vi "RemotePanel.vi"(0 "Refresh":i32=250, 1 "Remote Path":path, 2 "Remote App":refnum<vi>, 3 "Local  VI":refnum<vi>) -> ()   [LabVIEW 2014]
panel:
  out "Label.Text":string
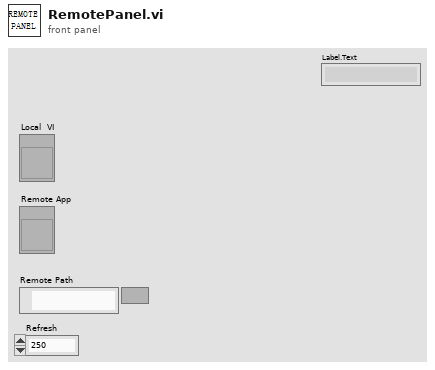
[diagram p1: front panel]
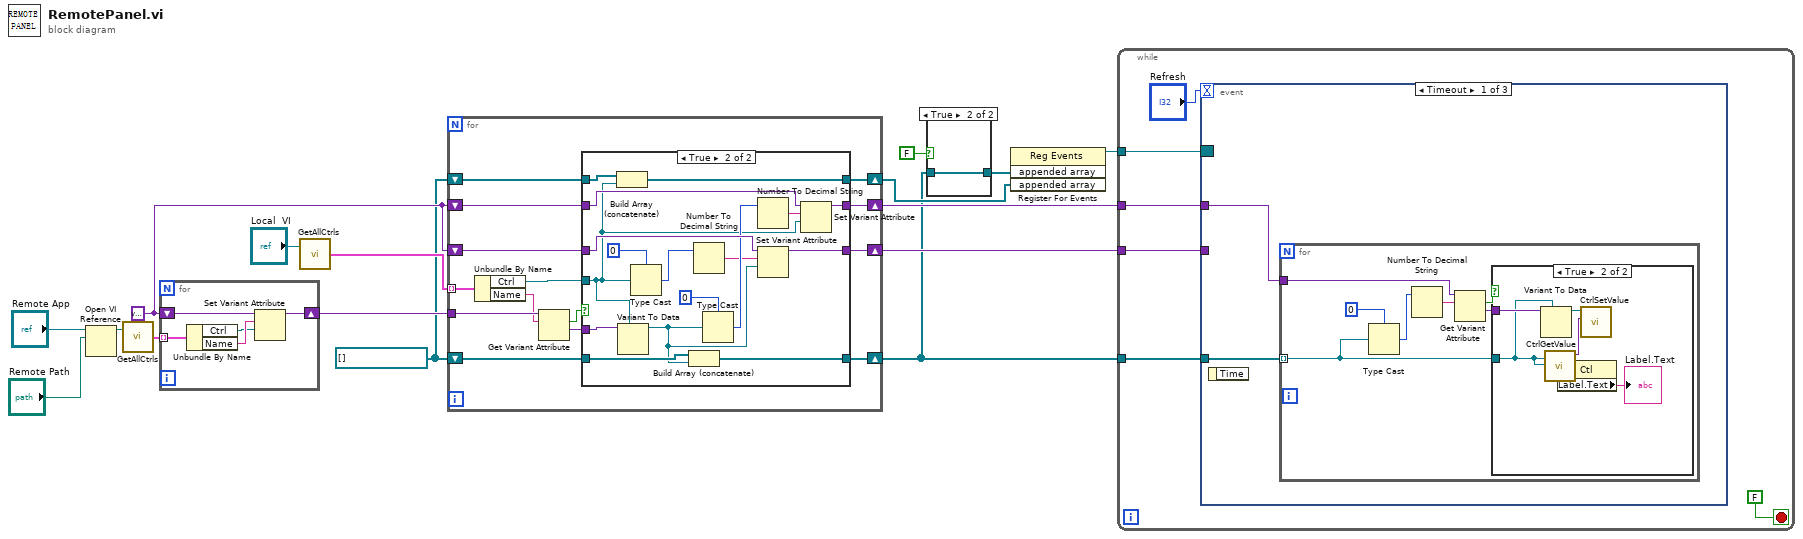
[diagram p0: block diagram]
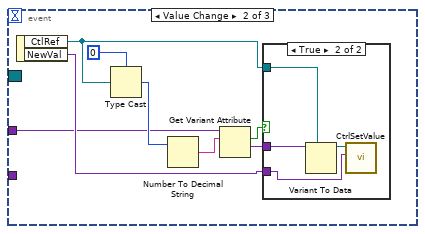
[diagram p5: hidden frame]
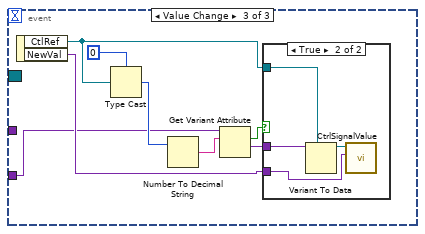
[diagram p7: hidden frame]
diagram:
  w9 = refnum<vi>[] [] ("appended array")
  w10 = variant ("variant")
  n1 = Open VI Reference(application reference (local)="Remote App", vi path="Remote Path") -> (vi reference=w13:refnum<vi>)  [unwired: 4 in, 1 out]
  n2 = call "GetAllCtrls.vi"("VI"=w13) -> ("Ctrls"=w14:cluster{"Name":string, "Ctrl":refnum<vi>}[])  [unwired: 1 in]
  n3 = for {
    tunnel: w14 -> [w21] mode=indexing
    shift-right: [w17] -> w11
    shift-left: w10 -> [w20]
    n4 = Unbundle By Name(w21) -> ("Ctrl"=w18:refnum<vi>, "Name"=w19:string)
    n5 = Set Variant Attribute(Variant=w20, name=w19, value=w18) -> (Variant out=w17:variant)  [unwired: 1 in, 2 out]
  }
  n6 = call "GetAllCtrls.vi"("VI"="Local  VI") -> ("Ctrls"=w12:cluster{"Name":string, "Ctrl":refnum<vi>}[])  [unwired: 1 in]
  n7 = for {
    tunnel: w12 -> [w35] mode=indexing
    shift-right: [w28] -> w7
    shift-left: w10 -> [w34]
    tunnel: w11 -> [w33]
    shift-right: [w29] -> w6
    shift-left: w10 -> [w30]
    shift-right: [w22] -> w8
    shift-left: w9 -> [w25]
    shift-right: [w23] -> w3
    shift-left: w9 -> [w24]
    n8 = Unbundle By Name(w35) -> ("Ctrl"=w27:refnum<vi>, "Name"=w32:string)
    n9 = Get Variant Attribute(Variant=w33, name=w32) -> (found=w31:bool, value=w26:variant)  [unwired: 2 in, 2 out]
    n10 = case shown="True" w31 {
      tunnel: w34 -> [w38 w56]
      tunnel: w30 -> [w39 w55]
      tunnel: [w39 w54] -> w29
      tunnel: [w38 w53] -> w28
      tunnel: w27 -> [_ w45]
      tunnel: w26 -> [_ w48]
      tunnel: w25 -> [w36 w44]
      tunnel: w24 -> [w37 w43]
      tunnel: [w37 w41] -> w23
      tunnel: [w36 w40] -> w22
      frame False {
      }
      frame True {
        n11 = Build Array (concatenate)(w44, w45) -> (w40:refnum<vi>[])
        n12 = Variant To Data(type=w45, Variant=w48) -> (data=w42:refnum<vi>)  [unwired: 1 in, 1 out]
        n13 = Type Cast(type=u32 0, x=w45) -> (*(type *) &x=w49:u32)
        n14 = Build Array (concatenate)(w43, w42) -> (w41:refnum<vi>[])
        n15 = Number To Decimal String(number=w49) -> (decimal integer string=w47:string)  [unwired: 1 in]
        n16 = Type Cast(type=u32 0, x=w42) -> (*(type *) &x=w51:u32)
        n17 = Number To Decimal String(number=w51) -> (decimal integer string=w46:string)  [unwired: 1 in]
        n18 = Set Variant Attribute(Variant=w55, name=w47, value=w42) -> (Variant out=w54:variant)  [unwired: 1 in, 2 out]
        n19 = Set Variant Attribute(Variant=w56, name=w46, value=w45) -> (Variant out=w53:variant)  [unwired: 1 in, 2 out]
      }
    }
  }
  n20 = case shown="True" FALSE {
    tunnel: w3 -> [_ w57]
    tunnel: [_ w57] -> w2
    frame False {
    }
    frame True {
    }
  }
  n21 = register-events(w2, w8) -> (reference out=w16:refnum<event-registration>)  [unwired: 2 in, 1 out]
  n22 = while {
    tunnel: w16 -> [w62]
    tunnel: w7 -> [w61]
    tunnel: w6 -> [w60]
    tunnel: w3 -> [w59]
    stop <- FALSE stop-if-true
    n23 = event shown="[0] Timeout" {
      selector: w62 -> [_ _ _]
      dyn-events: _ -> [_ _ _]
      timeout: "Refresh" -> [_ _ _]
      tunnel: w61 -> [w64 w78 _]
      tunnel: w60 -> [_ _ w90]
      tunnel: w59 -> [w65 _ _]
      event Timeout {
        n24 = event-data() -> ()  [unwired: 1 in, 1 out]
        n25 = for {
          tunnel: w65 -> [w66] mode=indexing
          tunnel: w64 -> [w67]
          n26 = Type Cast(type=u32 0, x=w66) -> (*(type *) &x=w71:u32)
          n27 = Number To Decimal String(number=w71) -> (decimal integer string=w70:string)  [unwired: 1 in]
          n28 = Get Variant Attribute(Variant=w67, name=w70) -> (found=w69:bool, value=w68:variant)  [unwired: 2 in, 2 out]
          n29 = case shown="True" w69 {
            tunnel: w68 -> [_ w77]
            tunnel: w66 -> [_ w74]
            frame False {
            }
            frame True {
              n30 = Variant To Data(type=w74, Variant=w77) -> (data=w76:refnum<vi>)  [unwired: 1 in, 1 out]
              n31 = call "CtrlGetValue.vi"("reference"=w74) -> ("variant"=w75:variant)  [unwired: 1 in, 3 out]
              n32 = property class="Ctl"(reference=w74) -> ("Label.Text"=→"Label.Text":string)  [unwired: 1 in, 2 out]
              n33 = call "CtrlSetValue.vi"("variant"=w75, "reference"=w76) -> ()  [unwired: 2 in, 1 out]
            }
          }
        }
      }
      event Value Change {
        n34 = event-data() -> ("CtlRef"=w80:refnum<vi>, "NewVal"=w79:variant)  [unwired: 1 in]
        n35 = Type Cast(type=u32 0, x=w80) -> (*(type *) &x=w84:u32)
        n36 = Number To Decimal String(number=w84) -> (decimal integer string=w83:string)  [unwired: 1 in]
        n37 = Get Variant Attribute(Variant=w78, name=w83) -> (found=w82:bool, value=w81:variant)  [unwired: 2 in, 2 out]
        n38 = case shown="True" w82 {
          tunnel: w81 -> [_ w89]
          tunnel: w80 -> [_ w88]
          tunnel: w79 -> [_ w86]
          frame False {
          }
          frame True {
            n39 = Variant To Data(type=w88, Variant=w89) -> (data=w87:refnum<vi>)  [unwired: 1 in, 1 out]
            n40 = call "CtrlSetValue.vi"("variant"=w86, "reference"=w87) -> ()  [unwired: 2 in, 1 out]
          }
        }
      }
      event Value Change {
        n41 = event-data() -> ("CtlRef"=w92:refnum<vi>, "NewVal"=w91:variant)  [unwired: 1 in]
        n42 = Type Cast(type=u32 0, x=w92) -> (*(type *) &x=w96:u32)
        n43 = Number To Decimal String(number=w96) -> (decimal integer string=w95:string)  [unwired: 1 in]
        n44 = Get Variant Attribute(Variant=w90, name=w95) -> (found=w94:bool, value=w93:variant)  [unwired: 2 in, 2 out]
        n45 = case shown="True" w94 {
          tunnel: w93 -> [_ w101]
          tunnel: w92 -> [_ w100]
          tunnel: w91 -> [_ w98]
          frame False {
          }
          frame True {
            n46 = Variant To Data(type=w100, Variant=w101) -> (data=w99:refnum<vi>)  [unwired: 1 in, 1 out]
            n47 = call "CtrlSignalValue.vi"("variant"=w98, "reference"=w99) -> ()  [unwired: 2 in, 1 out]
          }
        }
      }
    }
  }
